vi "0 to 999 to string sub vi.vi"() -> ()   [LabVIEW 2020]
panel:
  out "String":string
  in  "Numeric":dbl
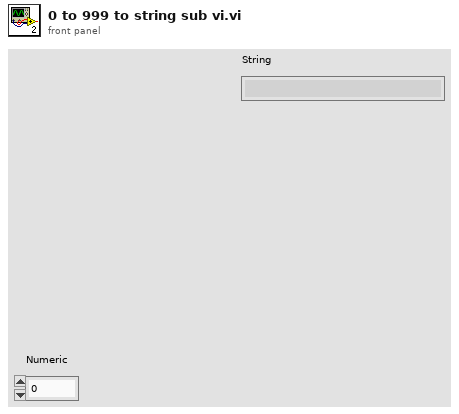
[diagram p1: front panel]
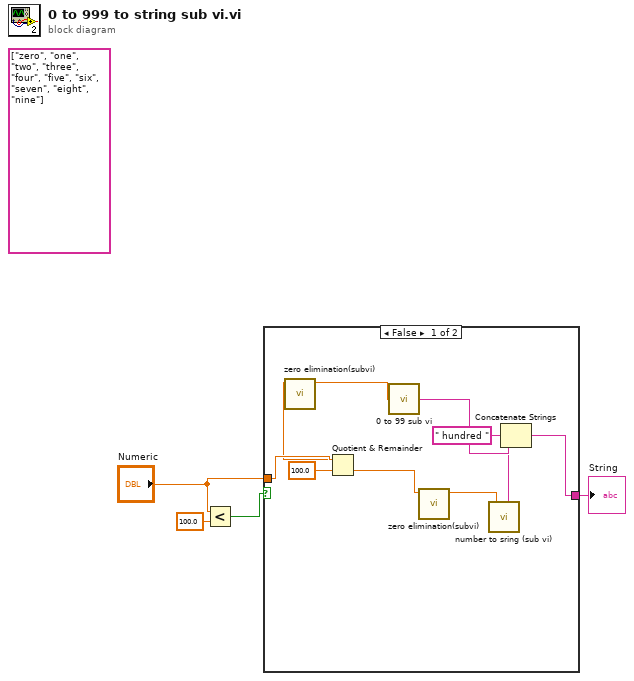
[diagram p0: block diagram]
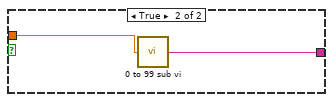
[diagram p2: hidden frame]
diagram:
  (unwired) string[] ["zero", "one", "two", "three", "four", "five", "six", "seven", "eight", "nine"]
  n1 = Less?(x="Numeric", y=100.0) -> (x < y?=w3:bool)
  n2 = case shown="False" w3 {
    tunnel: "Numeric" -> [w13 w16]
    tunnel: [w10 w15] -> w1
    frame False {
      n3 = Quotient & Remainder(x=w13, y=100.0) -> (x-y*floor(x/y)=w6:dbl, floor(x/y)=w9:dbl)
      n4 = call "zero elimination(subvi).vi"("Numeric"=w6) -> ("t"=w5:dbl)  [unwired: 10 in]
      n5 = call "0 to 99 sub vi.vi"("Numeric"=w5) -> ("String"=w8:string)
      n6 = call "zero elimination(subvi).vi"("Numeric"=w9) -> ("t"=w11:dbl)  [unwired: 10 in]
      n7 = call "number to sring (sub vi).vi"("Numeric"=w11) -> ("element"=w7:string)
      n8 = Concatenate Strings(w7, " hundred " ("string"), w8) -> (w10:string)
    }
    frame True {
      n9 = call "0 to 99 sub vi.vi"("Numeric"=w16) -> ("String"=w15:string)
    }
  }
  "String" <- w1
